vi "RC_Client 1.vi"(8 "error in (no error)":errorcluster, 11 "RC Type":T1) -> (0 "error out":errorcluster)   [LabVIEW 2016, in "RemoteControl.lvclass"]
uses:
  RemoteControl.lvclass
  Typedefs/RC Com Type--enum.ctl
  <userlib>/_OpenG.lib/numeric/numeric.llb/Random Number Within Range - I32__ogtk.vi
  <userlib>/_OpenG.lib/error/error.llb/Filter Error Codes (Array)__ogtk.vi
panel:
  in  "milliseconds to wait":u32
  out "time (1 message) (ms)":u32
  out "startup time (ms)":u32
  out "messsages/s":dbl
  in  "remote port":u16=6341
  in  "address":string
  out "Data":variant
  out "Messages":i32
  in  "Stop":bool
  out "Command reponse":string
  out "Command":string
  out "meta data\n(available commands)":string
  # "CLIENT (API)"
  # "Connection info"
  # "Message Sent"
  # "Message Received"
  # "Metrics"
  # "1"
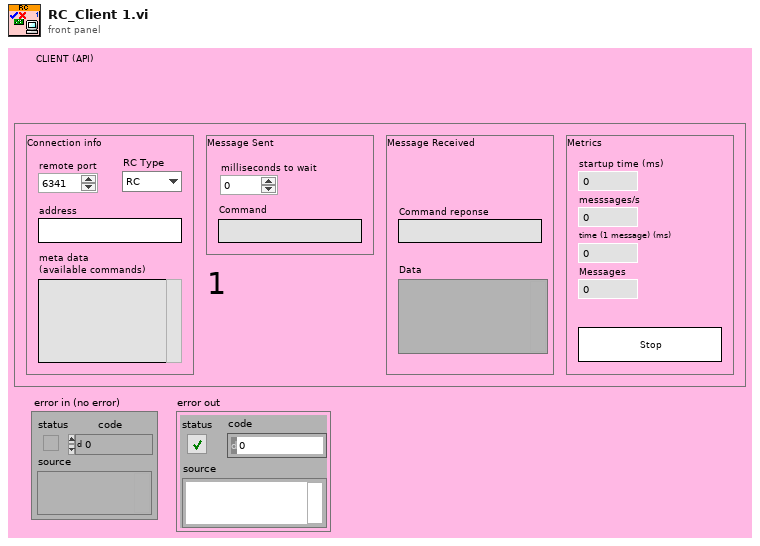
[diagram p1: front panel]
types:
  T1 = typedef "RemoteControl.lvclass/RC Com Type--enum.ctl" = enum16{"RC", "STM", "ZMQ"}
  T2 = cluster{"Command out":string, "Data out":variant, i32}
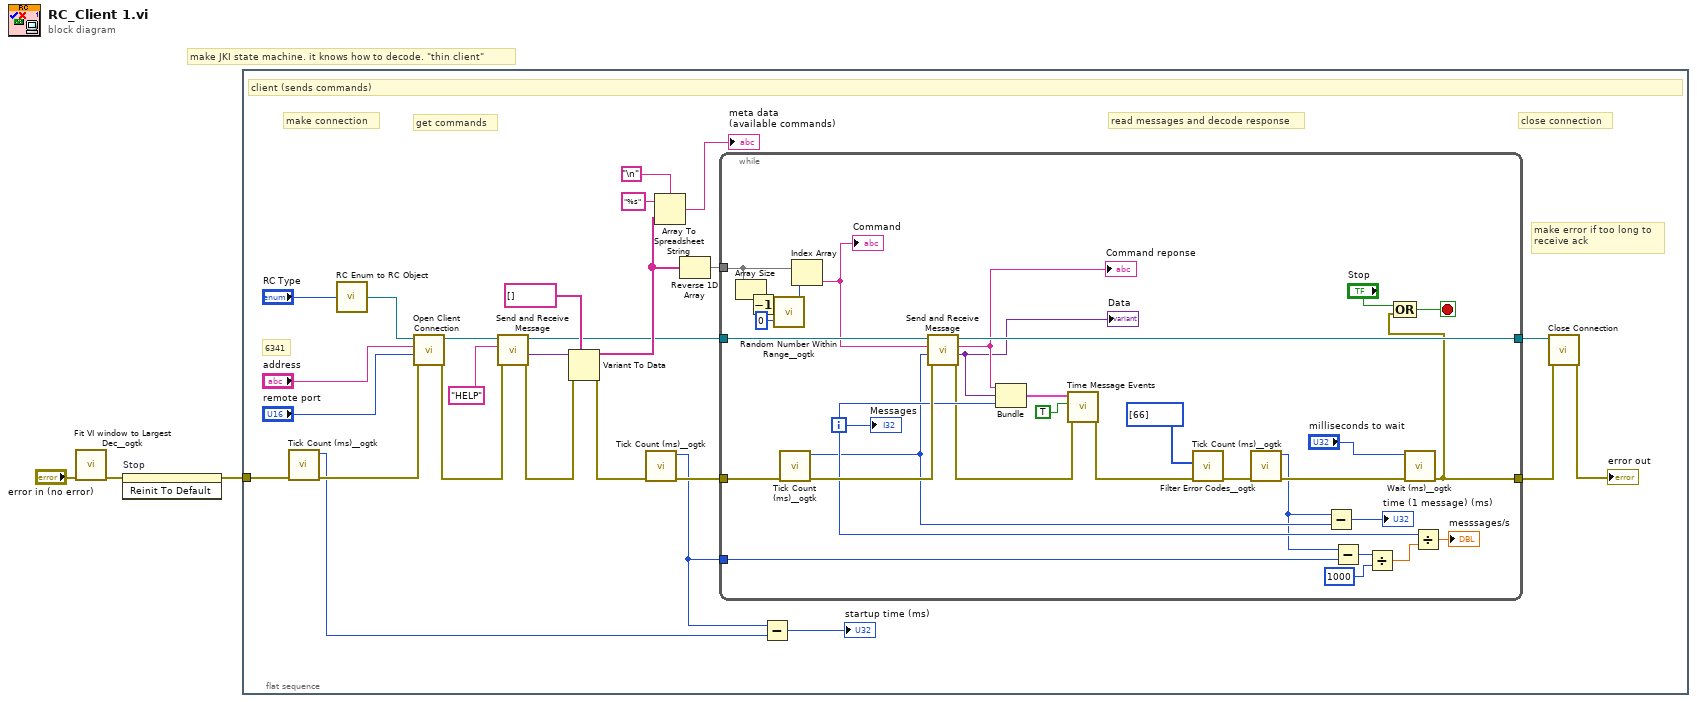
[diagram p0: block diagram]
diagram:
  # "make JKI state machine. it knows how to decode. \"thin client\""
  n1 = call <userlib>:"Fit VI window to Largest Dec__ogtk.vi"("error in (no error)"="error in (no error)") -> ("error out"=w3:errorcluster)  [unwired: 5 in, 1 out]
  n2 = invoke on="Stop" class="Bool" method="Reinit To Default"(error in=w3) -> (error out=w2:errorcluster)  [unwired: 2 in, 2 out]
  n3 = flat-sequence {
    tunnel: w2 -> [w15]
    frame #0 {
      # "close connection"
      # "read messages and decode response"
      # "get commands"
      # "make connection"
      # "6341"
      # "make error if too long to\nreceive ack"
      # "client (sends commands)"
      n4 = call <userlib>:"Tick Count (ms)__ogtk.vi"("error in (no error)"=w15) -> ("error out"=w24:errorcluster, "millisecond timer value"=w21:u32)  [unwired: 9 in]
      n5 = call "RC Enum to RC Object.vi"("RC Type"="RC Type") -> ("RemoteControl out"=w4:refnum<class "RemoteControl.lvclass">)
      n6 = call-dynamic "Open Client Connection.vi"("error in (no error)"=w24, "Port"="remote port", "address"="address", "RemoteControl in"=w4) -> ("error out"=w14:errorcluster, "RemoteControl out"=w12:refnum<class "RemoteControl.lvclass">)  [unwired: 6 in]
      n7 = call-dynamic "Send and Receive Message.vi"("error in (no error)"=w14, "Command"="HELP", "RemoteControl in"=w12) -> ("error out"=w8:errorcluster, "Data out"=w10:variant, "RemoteControl out"=w6:refnum<class "RemoteControl.lvclass">)  [unwired: 5 in, 1 out]
      n8 = Variant To Data(error in=w8, type=string[] [], Variant=w10) -> (data=w11:string[], error out=w7:errorcluster)
      n9 = call <userlib>:"Tick Count (ms)__ogtk.vi"("error in (no error)"=w7) -> ("error out"=w23:errorcluster, "millisecond timer value"=w16:u32)  [unwired: 9 in]
      n10 = Array To Spreadsheet String(delimiter (Tab)="\n", array=w11, 3:"%s" ("format string")) -> (spreadsheet string=→"meta data\n(available commands)":string)
      n11 = Reverse 1D Array(array=w11) -> (reversed array=w25:string[])
      n12 = while {
        tunnel: [w38] -> w29
        tunnel: [w58] -> w28
        tunnel: w23 -> [w53]
        tunnel: w6 -> [w59]
        tunnel: w25 -> [w42]
        tunnel: w16 -> [w32]
        i -> [w50]
        stop <- w61 stop-if-true
        n13 = Array Size(array=w42) -> (size(s)=w43:i32)
        n14 = Decrement(x=w43) -> (x-1=w41:i32)
        n15 = call-poly <userlib>:"Random Number Within Range__ogtk.vi"("High"=w41, "Low"=0) -> ("Random Number"=w45:i32)  [unwired: 3 in]
        n16 = call <userlib>:"Tick Count (ms)__ogtk.vi"("error in (no error)"=w53) -> ("error out"=w52:errorcluster, "millisecond timer value"=w39:u32)  [unwired: 9 in]
        n17 = Index Array(array=w42, index=w45) -> (element=w54:string)
        "Command" <- w54
        n18 = call-dynamic "Send and Receive Message.vi"("error in (no error)"=w52, "Data"=w39, "Command"=w54, "RemoteControl in"=w59) -> ("error out"=w40:errorcluster, "Data out"=w30:variant, "Command out"=w51:string, "RemoteControl out"=w58:refnum<class "RemoteControl.lvclass">)  [unwired: 4 in]
        "Command reponse" <- w51
        "Data" <- w30
        n19 = Bundle("Command out"=w51, "Data out"=w30, w50) -> (w49:T2)  [unwired: 1 in]
        n20 = call "Time Message Events.vi"("error in (no error)"=w40, "Debug Mode"=TRUE, "Message in"=w49) -> ("error out"=w31:errorcluster)  [unwired: 6 in, 2 out]
        n21 = call-poly <userlib>:"Filter Error Codes__ogtk.vi"("Error In"=w31, "Error Codes to Filter"=i32[] [66]) -> ("Error Out"=w57:errorcluster)  [unwired: 7 in, 2 out]
        n22 = call <userlib>:"Tick Count (ms)__ogtk.vi"("error in (no error)"=w57) -> ("error out"=w47:errorcluster, "millisecond timer value"=w34:u32)  [unwired: 9 in]
        n23 = Subtract(x=w34, y=w39) -> (x-y=→"time (1 message) (ms)":u32)
        n24 = Subtract(x=w34, y=w32) -> (x-y=w33:u32)
        n25 = Divide(x=w33, y=u32 1000) -> (x/y=w56:dbl)
        n26 = call <userlib>:"Wait (ms)__ogtk.vi"("error in (no error)"=w47, "milliseconds to wait"="milliseconds to wait") -> ("error out"=w38:errorcluster)  [unwired: 8 in, 1 out]
        n27 = Compound Arithmetic op=OR("Stop", w38) -> (w61:bool)
        n28 = Divide(x=w50, y=w56) -> (x/y=→"messsages/s":dbl)
        "Messages" <- w50
      }
      n29 = Subtract(x=w16, y=w21) -> (x-y=→"startup time (ms)":u32)
      n30 = call-dynamic "Close Connection.vi"("error in (no error)"=w29, "RemoteControl in"=w28) -> ("error out"=→"error out":errorcluster)  [unwired: 8 in, 1 out]
    }
  }
